vi "Command-Line Parse All.vi"() -> (0 "numeric keys":cluster{"key":string, "value":dbl}[](array[cluster]), 1 "boolean keys":cluster{"key":string, "value":bool}[](array[cluster]), 2 "string keys":cluster{"key":string, "value":string}[](array[cluster]), 3 "arguments":string[](array[string]), 4 "options":string[](array[string]), 5 "# arguments":i32)   [LabVIEW 2014]
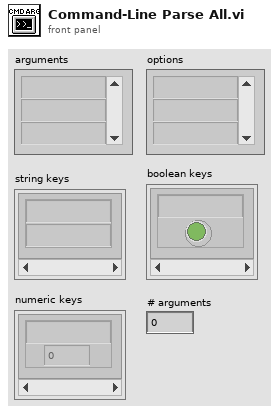
[diagram p1: front panel]
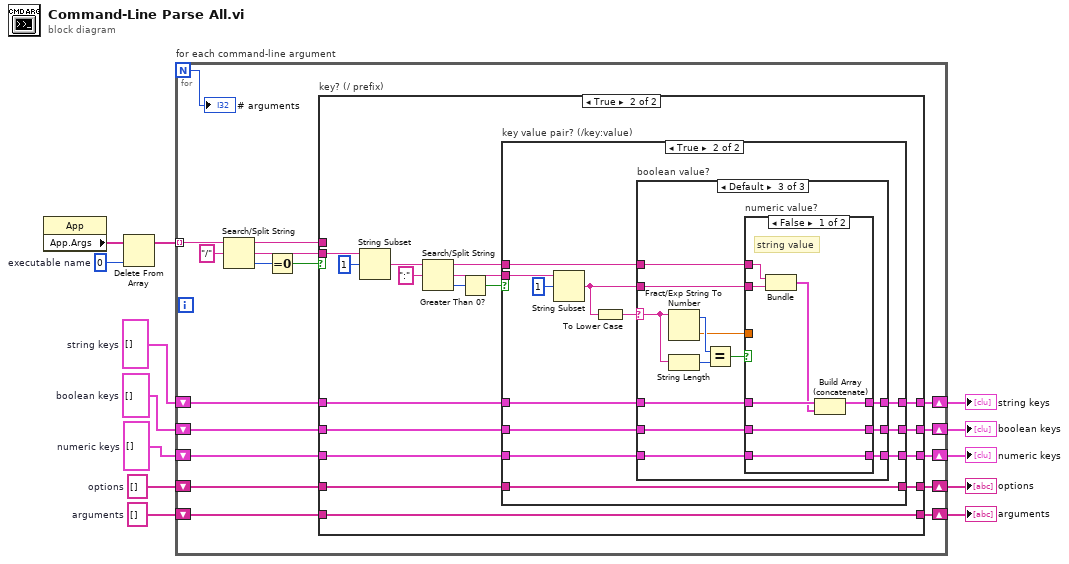
[diagram p0: block diagram]
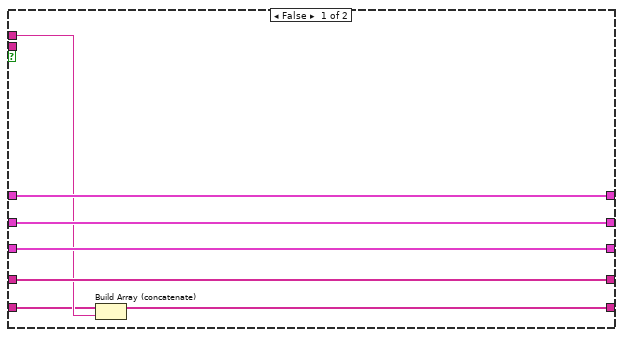
[diagram p2: hidden frame]
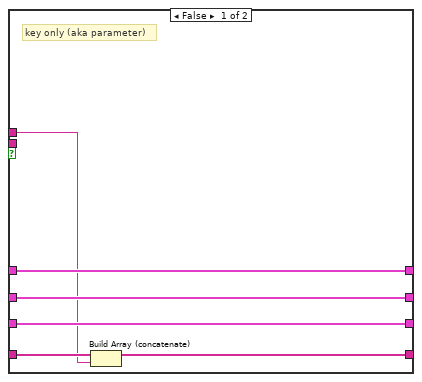
[diagram p3: hidden frame]
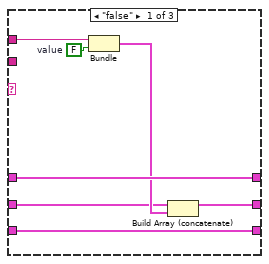
[diagram p4: hidden frame]
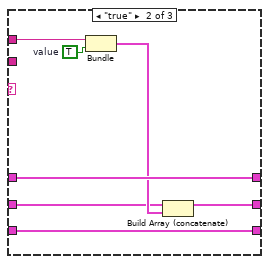
[diagram p5: hidden frame]
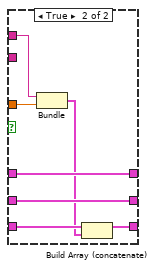
[diagram p6: hidden frame]
diagram:
  w7 = string[] []  # arguments
  w8 = string[] []  # options
  w9 = cluster{"key":string, "value":dbl}[] []  # numeric keys
  w10 = cluster{"key":string, "value":bool}[] []  # boolean keys
  w11 = cluster{"key":string, "value":string}[] []  # string keys
  w13 = 0  # executable name
  n1 = property class="App"() -> ("App.Args"=w1:string[])  [unwired: 2 in, 2 out]
  n2 = Delete From Array(array=w1, index=w13) -> (array with subset deleted=w12:string[])  [unwired: 1 in, 1 out]
  n3 = for "for each command-line argument" {
    N -> [w26]
    tunnel: w12 -> [w30] mode=indexing
    shift-right: [w22] -> w6
    shift-left: w11 -> [w23]
    shift-right: [w20] -> w5
    shift-left: w10 -> [w21]
    shift-right: [w17] -> w4
    shift-left: w9 -> [w24]
    shift-right: [w18] -> w3
    shift-left: w8 -> [w19]
    shift-right: [w15] -> w2
    shift-left: w7 -> [w16]
    n4 = Search/Split String(string=w30, search string/char (-)="/") -> (substring before match=w14:string, match + rest of string=w25:string, offset of match=w28:i32)  [unwired: 1 in]
    n5 = Equal To 0?(x=w28) -> (x = 0?=w27:bool)
    n6 = case "key? (/ prefix)" shown="True" w27 {
      tunnel: w25 -> [_ w54]
      tunnel: w24 -> [w35 w46]
      tunnel: [w35 w45] -> w17
      tunnel: w23 -> [w37 w44]
      tunnel: [w37 w43] -> w22
      tunnel: w21 -> [w36 w42]
      tunnel: [w36 w41] -> w20
      tunnel: w19 -> [w34 w39]
      tunnel: [w34 w40] -> w18
      tunnel: w16 -> [w31 w38]
      tunnel: [w33 w38] -> w15
      tunnel: w14 -> [w32 _]
      frame False {
        n7 = Build Array (concatenate)(w31, w32) -> (w33:string[])
      }
      frame True {
        n8 = String Subset(string=w54, offset (0)=1) -> (substring=w51:string)  [unwired: 1 in]
        n9 = Search/Split String(string=w51, search string/char (-)=":") -> (substring before match=w48:string, match + rest of string=w47:string, offset of match=w50:i32)  [unwired: 1 in]
        n10 = Greater Than 0?(x=w50) -> (x > 0?=w49:bool)
        n11 = case "key value pair? (/key:value)" shown="True" w49 {
          tunnel: w48 -> [w55 w69]
          tunnel: w47 -> [_ w71]
          tunnel: w46 -> [w57 w68]
          tunnel: [w57 w67] -> w45
          tunnel: w44 -> [w58 w65]
          tunnel: [w58 w64] -> w43
          tunnel: w42 -> [w59 w63]
          tunnel: [w59 w62] -> w41
          tunnel: [w60 w61] -> w40
          tunnel: w39 -> [w56 w61]
          frame False {
            # "key only (aka parameter)"
            n12 = Build Array (concatenate)(w56, w55) -> (w60:string[])
          }
          frame True {
            n13 = String Subset(string=w71, offset (0)=1) -> (substring=w66:string)  [unwired: 1 in]
            n14 = To Lower Case(string=w66) -> (all lower case string=w70:string)
            n15 = case "boolean value?" shown="Default" w70 {
              selector: w70 -> [_ _ w97]
              tunnel: w69 -> [w78 w86 w94]
              tunnel: w68 -> [w75 w82 w88]
              tunnel: [w75 w82 w87] -> w67
              tunnel: w66 -> [_ _ w93]
              tunnel: w65 -> [w76 w83 w92]
              tunnel: [w76 w83 w91] -> w64
              tunnel: w63 -> [w73 w80 w90]
              tunnel: [w77 w84 w89] -> w62
              frame "false" {
                w79 = FALSE  # value
                n16 = Bundle(w78, "value"=w79) -> (w74:cluster{string, "value":bool})  [unwired: 1 in]
                n17 = Build Array (concatenate)(w73, w74) -> (w77:cluster{"key":string, "value":bool}[])
              }
              frame "true" {
                w85 = TRUE  # value
                n18 = Bundle(w86, "value"=w85) -> (w81:cluster{string, "value":bool})  [unwired: 1 in]
                n19 = Build Array (concatenate)(w80, w81) -> (w84:cluster{"key":string, "value":bool}[])
              }
              frame Default {
                n20 = Fract/Exp String To Number(string=w97) -> (offset past number=w98:i32, number=w95:dbl)  [unwired: 3 in]
                n21 = String Length(string=w97) -> (length=w99:i32)
                n22 = Equal?(x=w98, y=w99) -> (x = y?=w96:bool)
                n23 = case "numeric value?" shown="False" w96 {
                  tunnel: w95 -> [_ w113]
                  tunnel: w94 -> [w106 w112]
                  tunnel: w93 -> [w105 _]
                  tunnel: w92 -> [w101 w111]
                  tunnel: [w104 w111] -> w91
                  tunnel: w90 -> [w103 w110]
                  tunnel: [w103 w110] -> w89
                  tunnel: w88 -> [w102 w108]
                  tunnel: [w102 w109] -> w87
                  frame False {
                    # "string value"
                    n24 = Bundle(w106, w105) -> (w100:cluster{string, string})  [unwired: 1 in]
                    n25 = Build Array (concatenate)(w101, w100) -> (w104:cluster{"key":string, "value":string}[])
                  }
                  frame True {
                    n26 = Bundle(w112, w113) -> (w107:cluster{string, dbl})  [unwired: 1 in]
                    n27 = Build Array (concatenate)(w108, w107) -> (w109:cluster{"key":string, "value":dbl}[])
                  }
                }
              }
            }
          }
        }
      }
    }
    "# arguments" <- w26
  }
  "numeric keys" <- w4
  "string keys" <- w6
  "boolean keys" <- w5
  "options" <- w3
  "arguments" <- w2
